vi "team_name.vi"(8 "error in (no error)":errorcluster, 11 "Igor in":refnum<class "Igor.lvclass">) -> (0 "error out":errorcluster, 2 "teamName":string, 3 "Igor out":refnum<class "Igor.lvclass">)   [LabVIEW 2015, in "Igor.lvclass"]
doc: "Created by Artem Shevelev\nshevelev.pro\nartem@shevelev.pro\nLabVIEW Portal: https://labviewportal.org/memberlist.php?mode=viewprofile&u=2340"
uses:
  Igor.lvclass
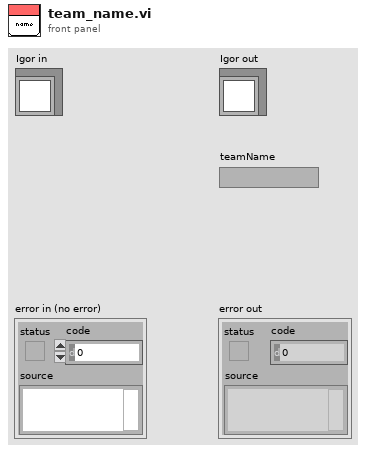
[diagram p1: front panel]
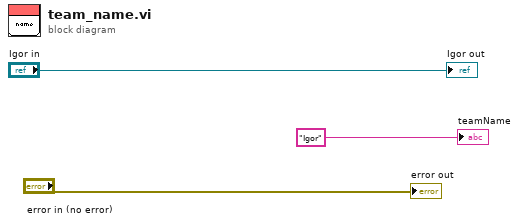
[diagram p0: block diagram]
diagram:
  "error out" <- "error in (no error)"
  "Igor out" <- "Igor in"
  "teamName" <- "Igor" ("teamName")
